vi "Derivada_numerica.vi"(9 "Funcion":dbl[](array[numeric]), 10 "Paso":dbl, 11 "Tiempo":dbl) -> (3 "Derivada":dbl[](array[numeric]))   [LabVIEW 2011]
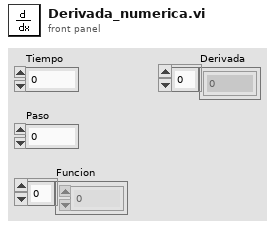
[diagram p1: front panel]
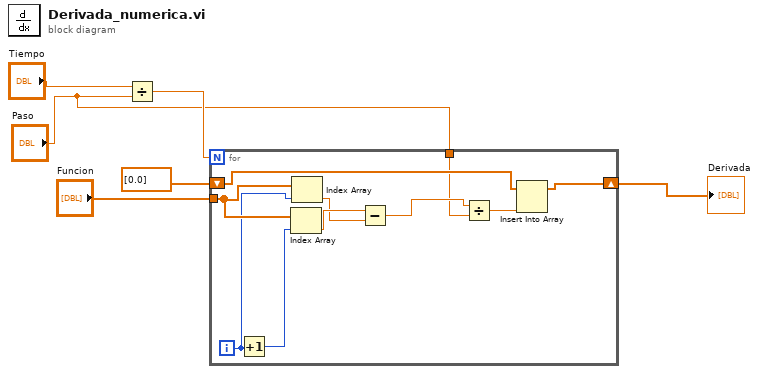
[diagram p0: block diagram]
diagram:
  n1 = Divide(x="Tiempo", y="Paso") -> (x/y=w4:dbl)
  n2 = for {
    N: w4 -> [_]
    tunnel: "Funcion" -> [w16]
    shift-right: [w14] -> w6
    shift-left: dbl[] [0.0] -> [w15]
    tunnel: "Paso" -> [w7]
    i -> [w9]
    n3 = Increment(x=w9) -> (x+1=w8:i32)
    n4 = Index Array(array=w16, index=w8) -> (element=w12:dbl)
    n5 = Index Array(array=w16, index=w9) -> (element=w11:dbl)
    n6 = Subtract(x=w12, y=w11) -> (x-y=w10:dbl)
    n7 = Divide(x=w10, y=w7) -> (x/y=w13:dbl)
    n8 = Insert Into Array(array=w15, new element=w13) -> (w14:dbl[])  [unwired: 1 in]
  }
  "Derivada" <- w6
